vi "test_daq_caller.vi"() -> ()   [LabVIEW 2018]
panel:
  out "Outputs":T1(array[cluster])
  in  "Requests":string[](array[string])
  out "error out":errorcluster
  in  "error in":errorcluster
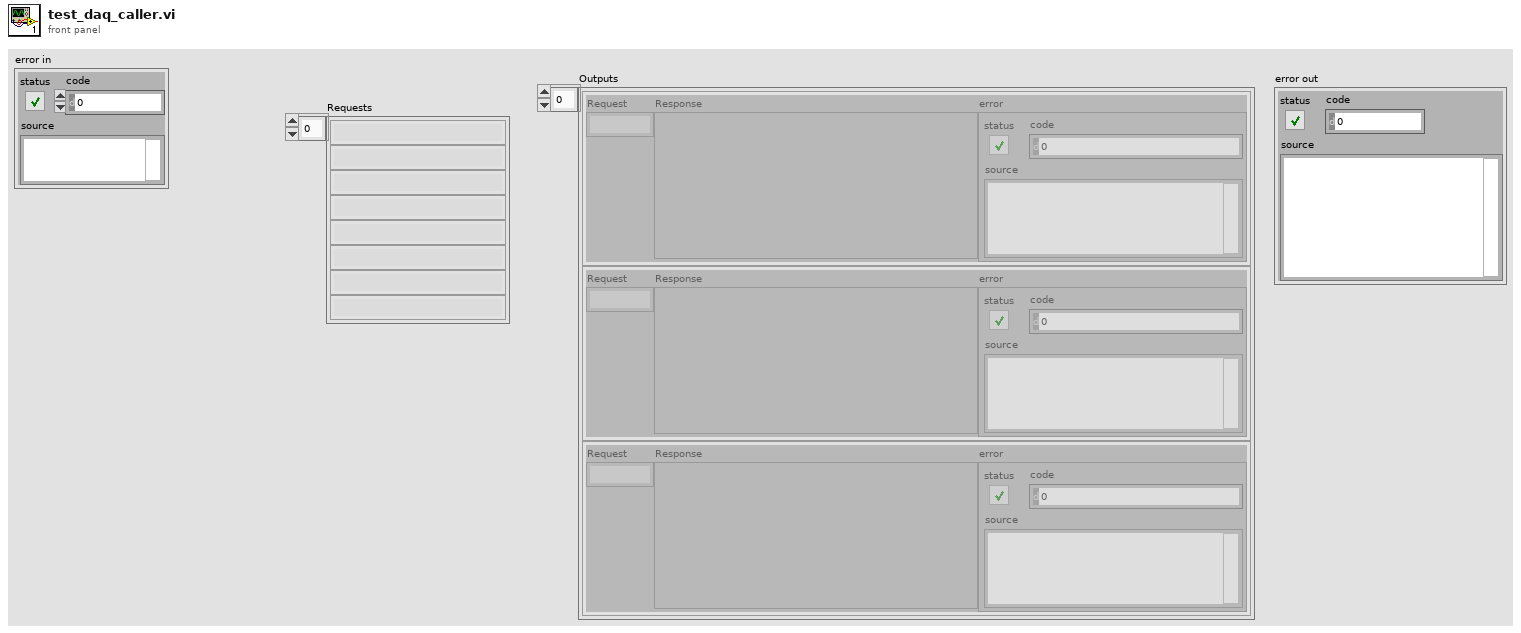
[diagram p1: front panel]
types:
  T1 = cluster{"Request":string, "Response":variant, "error":errorcluster}[]
  T2 = cluster{"Request":string, "Response":variant, "error":errorcluster}
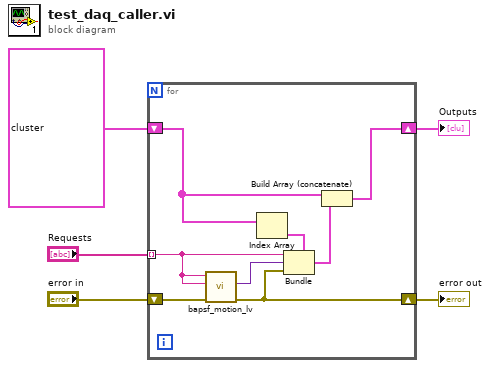
[diagram p0: block diagram]
diagram:
  n1 = for {
    tunnel: "Requests" -> [w9] mode=indexing
    shift-right: [w7] -> w4
    shift-left: "error in" -> [w13]
    shift-right: [w6] -> w1
    shift-left: T1 [{"Request"="", "Response"=variant, "error"={"status"=TRUE, "code"=0, "source"=""}}] -> [w11]
    n2 = call "bapsf_motion_lv.vi"("error in"=w13, "Request data"=w9, "Request"=w9) -> ("error out"=w7:errorcluster, "Response data"=w8:variant)  [unwired: 3 in]
    n3 = Index Array(array=w11) -> (element=w10:T2)  [unwired: 1 in]
    n4 = Bundle(cluster=w10, "Request"=w9, "Response"=w8, "error"=w7) -> (w12:T2)
    n5 = Build Array (concatenate)(w11, w12) -> (w6:T1)
  }
  "error out" <- w4
  "Outputs" <- w1
